vi "RS232 Communication Code.vi"() -> ()   [LabVIEW 2022 SP3]
uses:
  <vilib>/Instr/_visa.llb/VISA Configure Serial Port (Instr).vi
panel:
  out "read buffer":string
  in  "write buffer":string
  in  "stop":bool
  in  "baud rate (9600)":u32=9600
  in  "VISA resource name":refnum<visa-resource-name>
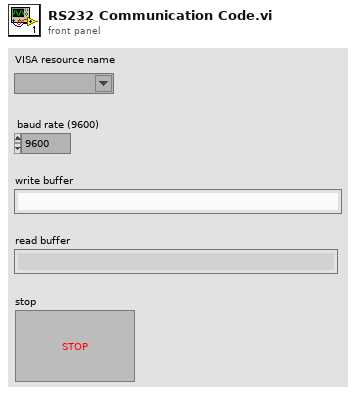
[diagram p1: front panel]
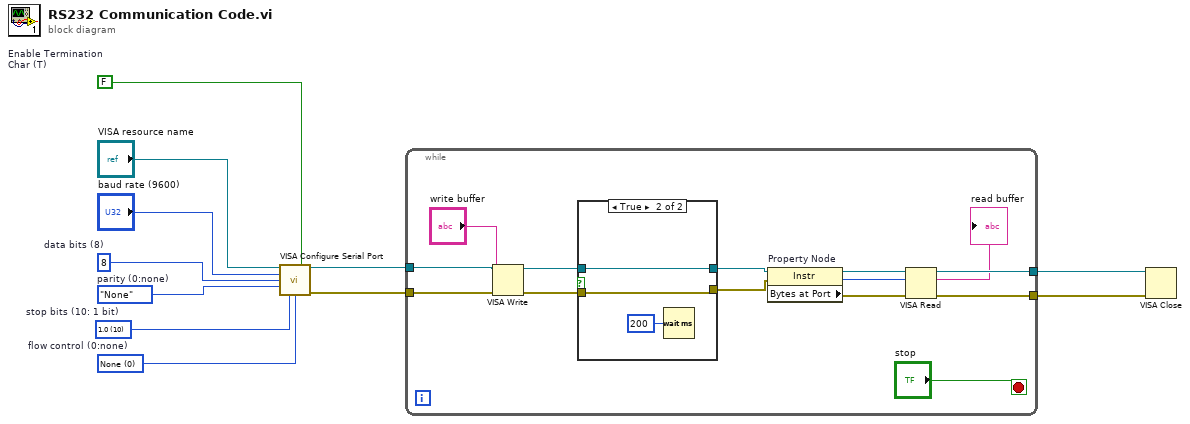
[diagram p0: block diagram]
diagram:
  w5 = FALSE  # Enable Termination Char (T)
  w6 = u16 0 items=["None", "XON/XOFF", "RTS/CTS", "XON/XOFF & RTS/CTS", "DTR/DSR", "XON/XOFF & DTR/DSR"]  # flow control (0:none)
  w7 = u16 10 items=["1.0"=10, "1.5"=15, "2.0"=20]  # stop bits (10: 1 bit)
  w8 = enum16{"None", "Odd", "Even", "Mark", "Space"}."None"  # parity (0:none)
  w9 = u16 8  # data bits (8)
  n1 = call-poly "VISA Configure Serial Port"("VISA resource name"="VISA resource name", "Enable Termination\nChar (T)"=w5, "baud rate (9600)"="baud rate (9600)", "data bits (8)"=w9, "parity (0:none)"=w8, "stop bits (10: 1 bit)"=w7, "flow control (0:none)"=w6) -> ("VISA resource name out"=w1:refnum<visa-resource-name>, "error out"=w3:errorcluster)  [unwired: 7 in]
  n2 = while {
    tunnel: [w24] -> w4
    tunnel: w3 -> [w23]
    tunnel: [w22] -> w2
    tunnel: w1 -> [w20]
    stop <- "stop" stop-if-true
    n3 = VISA Write(VISA resource name=w20, write buffer="write buffer", error in (no error)=w23) -> (VISA resource name out=w15:refnum<visa-resource-name>, error out=w13:errorcluster)  [unwired: 1 out]
    n4 = case shown="True" {
      selector: _ -> [_ _]
      tunnel: w15 -> [_ w28]
      tunnel: [_ w28] -> w14
      tunnel: w13 -> [_ w27]
      tunnel: [_ w27] -> w12
      frame False {
      }
      frame True {
        n5 = Wait (ms)(milliseconds to wait=u32 200) -> ()  [unwired: 1 out]
      }
    }
    n6 = property on="Property Node" class="Instr"(reference=w14, error in=w12) -> (reference out=w18:refnum<visa-resource-name>, error out=w16:errorcluster, "Bytes at Port"=w17:u32)
    n7 = VISA Read(VISA resource name=w18, byte count=w17, error in (no error)=w16) -> (VISA resource name out=w24:refnum<visa-resource-name>, read buffer=→"read buffer":string, error out=w22:errorcluster)  [unwired: 1 out]
  }
  n8 = VISA Close(VISA resource name=w4, error in (no error)=w2) -> ()  [unwired: 1 out]
